vi "_RS232_EEPROM_vna_jet.vi"(0 "VISA resource name":refnum<visa-resource-name>="COM3", 1 "Function":enum16{"Write to EEPROM", "Read From EEPROM"}(ring)=enum."Read From EEPROM", 2 "Select channel":u32, 3 "input_cmd":string="44 A0 00 01 02 03", 5 "Error in":errorcluster) -> (13 "readout":string[](array[string]), 14 "Duplicate VISA resource name":refnum<visa-resource-name>="COM1", 15 "readout":string, 16 "readout":u8[](array[numeric])=[3, 4, 33, 1, 0, 0, 4, 65, 132, 128, 213, 0, 103, 0, 0, 0, 0, 0, 1, 0, 72, 73, 83, 69, 84, 69, 67, 0, 0, 0, 0, 0, 0, 0, 0, 0, 0, 0, 0, 0, 76, 48, 48, 84, 72, 48, 48, 50, 45, 77, 49, 45, 82, 0, 0, 0, 65, 0, 0, 0, 1, 0, 0, 250, 0, 0, 0, 0, 49, 50, 51, 50, 55, 49, 48, 48, 48, 51, 0, 0, 0, 0, 0, 0, 49, 50, 49, 49, 50, 50, 0, 0, 0, 0, 0, 28, 72, 51, 67, 0, 0, 0, 0, 0, 0, 0, 0, 48, 52, 48, 52, 65, 49, 49, 50, 1, 2, 0, 1, 0, 0, 0, 0, 0, 0, 0, 0, 95, 0, 0, 0, 0, 0, 0, 0, 0, 0, 0, 0, 0, 0, 0, 0, 0, 0, 0, 0, 0, 0, 0, 0, 0, 0, 0, 0, 0, 0, 0, 0, 0, 0, 0, 0, 0, 0, 0, 0, 0, 0, 0, 0, 0, 0, 0, 0, 0, 0, 0, 0, 0, 0, 0, 0, 0, 0, 0, 0, 0, 0, 0, 0, 0, 0, 0, 0, 0, 0, 0, 0, 0, 0, 0, 0, 0, 0, 0, 0, 0, 0, 0, 0, 0, 0, 0, 0, 0, 0, 0, 0, 0, 0, 0, 0, 0, 0, 0, 0, 0, 0, 0, 0, 0, 0, 0, 0, 0, 0, 0, 0, 0, 0, 0, 0, 0, 0, 0, 0, 0, 0, 0, 0, 0, 0, 0, 0, 0] format="%x", 17 "Message":string="Read EEPROM", 18 "Result":bool=TRUE, 19 "error out":errorcluster={"status"=FALSE, "code"=1073676294, "source"="RS232-I2C-EEPROM.vi中的VISA读取"})   [LabVIEW 2011]
uses:
  <vilib>/Instr/_visa.llb/VISA Configure Serial Port (Instr).vi
panel:
  in  "Mode":u32(ring) items=["0~EasyI2C", "1~TimingI2C"]
  # "RS232-I2C Writting and Reading"
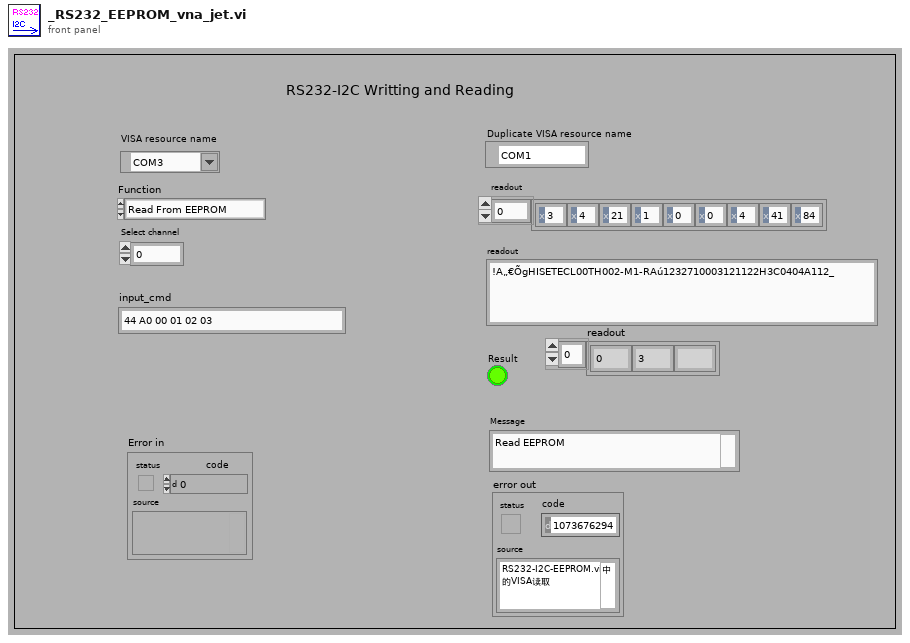
[diagram p1: front panel]
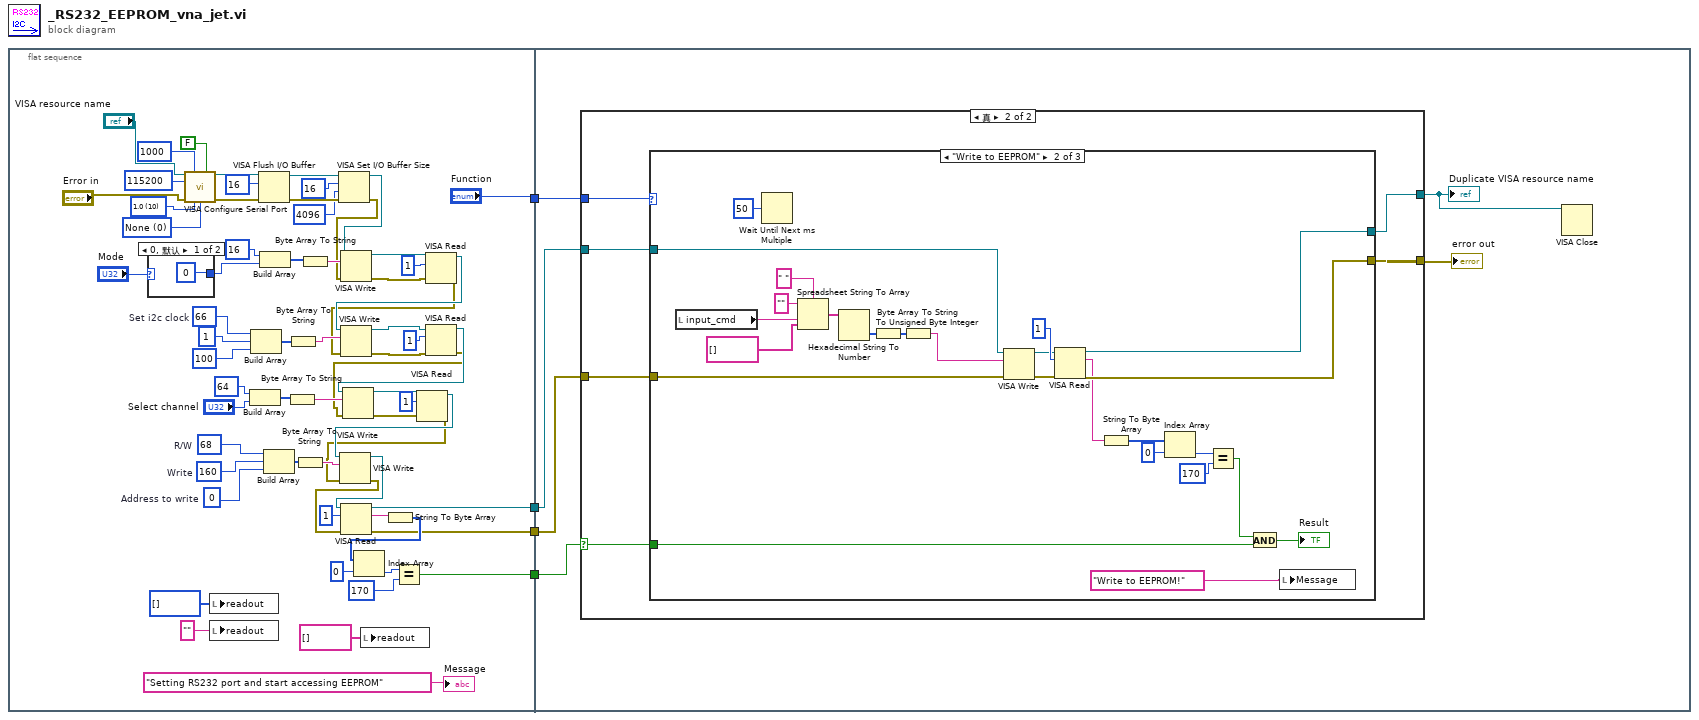
[diagram p0: block diagram]
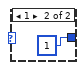
[diagram p2: hidden frame]
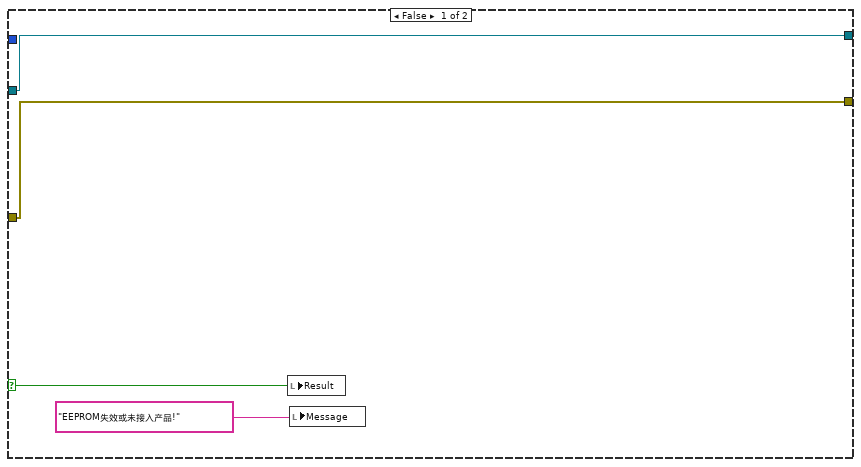
[diagram p3: hidden frame]
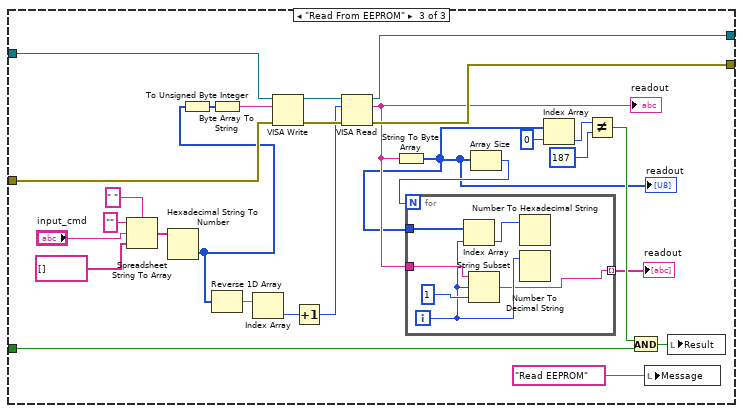
[diagram p5: hidden frame]
diagram:
  n1 = flat-sequence {
    tunnel: [w29] -> w4
    tunnel: [w28] -> w3
    tunnel: [w27] -> w2
    tunnel: ["Function"] -> w1
    tunnel: w4 -> [w78]
    tunnel: w3 -> [w77]
    tunnel: w2 -> [w76]
    tunnel: w1 -> [w75]
    frame #0 {
      w33 = u32 0  # Address to write
      w37 = u32 160  # Write
      w35 = u32 68  # R/W
      w50 = u32 66  # Set i2c clock
      w69 = u16 0 items=["None", "XON/XOFF", "RTS/CTS", "XON/XOFF & RTS/CTS", "DTR/DSR", "XON/XOFF & DTR/DSR"] ("flow control (0:none)")
      w63 = u16 10 items=["1.0"=10, "1.5"=15, "2.0"=20] ("stop bits (10: 1 bit)")
      n2 = case shown="0, 默认" "Mode" {
        tunnel: [u32 0 ("channel") u32 1 ("channel")] -> w56
        frame 0, Default {
        }
        frame 1 {
        }
      }
      n3 = call-poly "VISA Configure Serial Port"("VISA resource name"="VISA resource name", "timeout (10sec)"=u32 1000 ("timeout"), "Enable Termination\nChar (T)"=FALSE ("Enable Termination\nChar (T)"), "baud rate (9600)"=u32 115200 ("baud rate"), "error in (no error)"="Error in", "stop bits (10: 1 bit)"=w63, "flow control (0:none)"=w69) -> ("VISA resource name out"=w70:refnum<visa-resource-name>, "error out"=w43:errorcluster)  [unwired: 7 in]
      n4 = local write "readout"(u8[] [] ("readout")) -> ()
      n5 = local write "readout"("") -> ()
      n6 = Build Array(u32 64 ("size (0)"), "Select channel") -> (w54:u32[])
      n7 = Build Array(w50, u32 1 ("size (0)"), u32 100 ("size (0)")) -> (w49:u32[])
      n8 = VISA Flush I/O Buffer(VISA resource name=w70, mask (16)=u16 16, error in (no error)=w43) -> (VISA resource name out=w66:refnum<visa-resource-name>, error out=w65:errorcluster)
      n9 = Build Array(u32 16 ("size (0)"), w56) -> (w55:u32[])
      n10 = Build Array(w35, w37, w33) -> (w36:u32[])
      n11 = Byte Array To String(unsigned byte array=w54) -> (string=w46:string)
      n12 = Byte Array To String(unsigned byte array=w49) -> (string=w45:string)
      n13 = Byte Array To String(unsigned byte array=w36) -> (string=w40:string)
      n14 = Byte Array To String(unsigned byte array=w55) -> (string=w58:string)
      n15 = VISA Set I/O Buffer Size(VISA resource name=w66, mask (16)=u16 16, size (4096)=u32 4096 ("size (0)"), error in (no error)=w65) -> (VISA resource name out=w59:refnum<visa-resource-name>, error out=w42:errorcluster)
      n16 = VISA Write(VISA resource name=w59, write buffer=w58, error in (no error)=w42) -> (VISA resource name out=w22:refnum<visa-resource-name>, error out=w21:errorcluster)  [unwired: 1 out]
      n17 = local write "readout"(string[] [] ("readout")) -> ()
      n18 = VISA Read(VISA resource name=w22, byte count=u32 1, error in (no error)=w21) -> (VISA resource name out=w20:refnum<visa-resource-name>, error out=w17:errorcluster)  [unwired: 2 out]
      n19 = VISA Write(VISA resource name=w20, write buffer=w45, error in (no error)=w17) -> (VISA resource name out=w19:refnum<visa-resource-name>, error out=w16:errorcluster)  [unwired: 1 out]
      n20 = VISA Read(VISA resource name=w19, byte count=u32 1, error in (no error)=w16) -> (VISA resource name out=w18:refnum<visa-resource-name>, error out=w15:errorcluster)  [unwired: 2 out]
      n21 = VISA Write(VISA resource name=w18, write buffer=w46, error in (no error)=w15) -> (VISA resource name out=w14:refnum<visa-resource-name>, error out=w13:errorcluster)  [unwired: 1 out]
      n22 = VISA Read(VISA resource name=w14, byte count=u32 1, error in (no error)=w13) -> (VISA resource name out=w11:refnum<visa-resource-name>, error out=w10:errorcluster)  [unwired: 2 out]
      n23 = VISA Write(VISA resource name=w11, write buffer=w40, error in (no error)=w10) -> (VISA resource name out=w34:refnum<visa-resource-name>, error out=w41:errorcluster)  [unwired: 1 out]
      n24 = VISA Read(VISA resource name=w34, byte count=u32 1, error in (no error)=w41) -> (VISA resource name out=w28:refnum<visa-resource-name>, read buffer=w39:string, error out=w27:errorcluster)  [unwired: 1 out]
      n25 = String To Byte Array(string=w39) -> (unsigned byte array=w30:u8[])
      n26 = Index Array(array=w30, index=0) -> (element=w32:u8)
      n27 = Equal?(x=w32, y=u32 170 ("size (0)")) -> (x = y?=w29:bool)
      "Message" <- "Setting RS232 port and start accessing EEPROM" ("Message")
    }
    frame #1 {
      n28 = case shown="真" w78 {
        selector: w78 -> [w79 w85]
        tunnel: w77 -> [w81 w88]
        tunnel: w76 -> [w82 w87]
        tunnel: w75 -> [_ w86]
        tunnel: [w82 w84] -> w74
        tunnel: [w81 w83] -> w73
        frame False {
          n29 = local write "Result"(w79) -> ()
          n30 = local write "Message"("EEPROM失效或未接入产品!" ("message")) -> ()
        }
        frame True {
          n31 = case shown="\"Write to EEPROM\"" w86 {
            tunnel: w88 -> [w90 w115 w143]
            tunnel: w87 -> [w89 w114 w142]
            tunnel: [w90 w112 w139] -> w83
            tunnel: [w89 w113 w138] -> w84
            tunnel: w85 -> [_ w111 w133]
            frame Default {
            }
            frame "Write to EEPROM" {
              n32 = local read "input_cmd"() -> (w98:string)
              n33 = Wait Until Next ms Multiple(millisecond multiple=u32 50) -> ()  [unwired: 1 out]
              n34 = Spreadsheet String To Array(delimiter (Tab)=" " ("分隔符(Tab)"), format string="" ("格式字符串"), spreadsheet string=w98, array type (2D Dbl)=string[] [] ("数组")) -> (array=w95:string[])
              n35 = Hexadecimal String To Number(string=w95) -> (number=w96:u32[])  [unwired: 2 in, 1 out]
              n36 = To Unsigned Byte Integer(number=w96) -> (unsigned 8bit integer=w91:u8[])
              n37 = Byte Array To String(unsigned byte array=w91) -> (string=w92:string)
              n38 = VISA Write(VISA resource name=w115, write buffer=w92, error in (no error)=w114) -> (VISA resource name out=w104:refnum<visa-resource-name>, error out=w103:errorcluster)  [unwired: 1 out]
              n39 = VISA Read(VISA resource name=w104, byte count=u32 1, error in (no error)=w103) -> (VISA resource name out=w112:refnum<visa-resource-name>, read buffer=w102:string, error out=w113:errorcluster)  [unwired: 1 out]
              n40 = String To Byte Array(string=w102) -> (unsigned byte array=w101:u8[])
              n41 = Index Array(array=w101, index=0) -> (element=w100:u8)
              n42 = Equal?(x=w100, y=u32 170 ("size (0)")) -> (x = y?=w99:bool)
              n43 = And(x=w99, y=w111) -> (x .and. y?=→"Result":bool)
              n44 = local write "Message"("Write to EEPROM!" ("Message")) -> ()
            }
            frame "Read From EEPROM" {
              n45 = Spreadsheet String To Array(delimiter (Tab)=" " ("分隔符(Tab)"), format string="" ("格式字符串"), spreadsheet string="input_cmd", array type (2D Dbl)=string[] [] ("数组")) -> (array=w124:string[])
              n46 = Hexadecimal String To Number(string=w124) -> (number=w117:u32[])  [unwired: 2 in, 1 out]
              n47 = To Unsigned Byte Integer(number=w117) -> (unsigned 8bit integer=w121:u8[])
              n48 = Byte Array To String(unsigned byte array=w121) -> (string=w120:string)
              n49 = Reverse 1D Array(array=w117) -> (reversed array=w126:u32[])
              n50 = Index Array(array=w126) -> (element=w119:u32)  [unwired: 1 in]
              n51 = VISA Write(VISA resource name=w143, write buffer=w120, error in (no error)=w142) -> (VISA resource name out=w141:refnum<visa-resource-name>, error out=w140:errorcluster)  [unwired: 1 out]
              n52 = Increment(x=w119) -> (x+1=w116:u32)
              n53 = VISA Read(VISA resource name=w141, byte count=w116, error in (no error)=w140) -> (VISA resource name out=w139:refnum<visa-resource-name>, read buffer=w130:string, error out=w138:errorcluster)  [unwired: 1 out]
              "readout" <- w130
              n54 = String To Byte Array(string=w130) -> (unsigned byte array=w129:u8[])
              "readout" <- w129
              n55 = Array Size(array=w129) -> (size(s)=w137:i32)
              n56 = for {
                N: w137 -> [_]
                tunnel: w129 -> [w149]
                tunnel: w130 -> [w148]
                tunnel: [w144] -> w131 mode=indexing
                i -> [w145]
                n57 = Index Array(array=w149, index=w145) -> (element=w146:u8)
                n58 = String Subset(string=w148, offset (0)=w145, length (rest)=1 ("length (rest)")) -> (substring=w144:string)
                n59 = Number To Hexadecimal String(2:w146) -> ()  [unwired: 1 in, 1 out]
                n60 = Number To Decimal String(number=w145) -> ()  [unwired: 1 in, 1 out]
              }
              "readout" <- w131
              n61 = Index Array(array=w129, index=0) -> (element=w134:u8)
              n62 = Not Equal?(x=w134, y=u32 187 ("size (0)")) -> (x != y?=w132:bool)
              n63 = And(x=w132, y=w133) -> (x .and. y?=w128:bool)
              n64 = local write "Message"("Read EEPROM" ("Message")) -> ()
              n65 = local write "Result"(w128) -> ()
            }
          }
        }
      }
      "Duplicate VISA resource name" <- w73
      "error out" <- w74
      n66 = VISA Close(VISA resource name=w73) -> ()  [unwired: 1 in, 1 out]
    }
  }
